vi "From Lockin to Pulse .vi"(7 "Pulse Configuration in":T1={"Post-trigger delay"=0.01, "Post-trigger duration"=0.1, "Rate"=1000000.0, "Ranges"=[10.0], "Re-name channels"=[], "Active channels"="0:1", "External clock"=FALSE} {"Rate" format="%#_8pHz"; "Post-trigger duration" format="%#_6ps"; "Post-trigger delay" format="%#_6ps"; "Ranges" format="%#_6pV"}, 11 "Lockin Configuration in":T2={"Post-trigger delay"=0.01, "Post-trigger duration"=0.1, "Rate"=1000000.0, "Ranges"=[10.0], "Re-name channels"=[], "Active channels"="0:1", "External\nclock"=FALSE, "Frequencies"=[], "Time\nconstant"=1.0, "Output \namplitudes"=[], "Input\nchannles"=[]} {"Output \namplitudes" format="%#_6pV"; "Time\nconstant" format="%#_6ps"; "Frequencies" format="%#_6pHz"; "Rate" format="%#_8pHz"; "Post-trigger duration" format="%#_6ps"; "Post-trigger delay" format="%#_6ps"; "Ranges" format="%#_6pV"}) -> (3 "Pulse  Configuration out":T1={"Post-trigger delay"=0.01, "Post-trigger duration"=0.1, "Rate"=1000000.0, "Ranges"=[10.0], "Re-name channels"=[], "Active channels"="0:1", "External clock"=FALSE} {"Rate" format="%#_8pHz"; "Post-trigger duration" format="%#_6ps"; "Post-trigger delay" format="%#_6ps"; "Ranges" format="%#_6pV"})   [LabVIEW 2021]
uses:
  Pusle Driver Configuration.ctl
  Lockin Digitizer Driver/Lockin Digitizer Configuration.ctl
panel:
  # "Digitizer config"
  # "Lock-in config"
  # "#0\n\n#1"
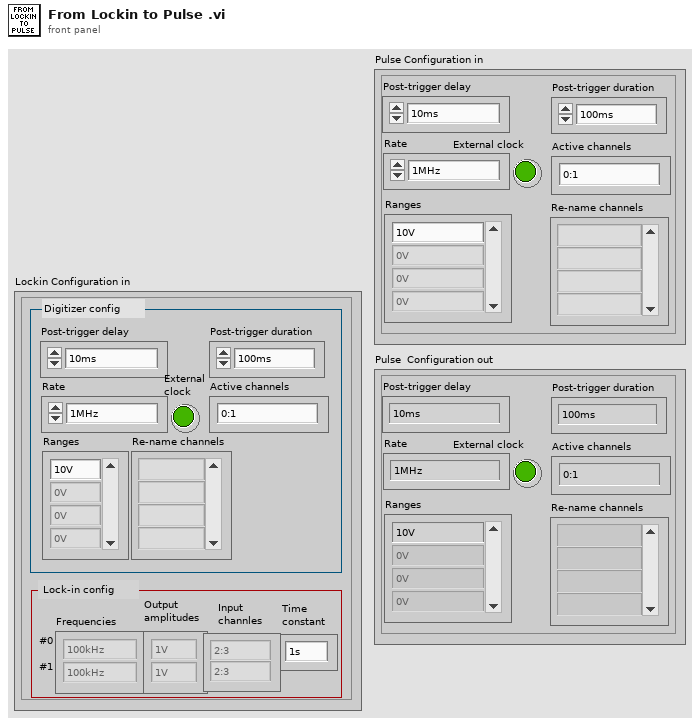
[diagram p1: front panel]
types:
  T1 = typedef "Pusle Driver Configuration.ctl" = cluster{"Post-trigger delay":dbl, "Post-trigger duration":dbl, "Rate":dbl, "Ranges":dbl[], "Re-name channels":string[], "Active channels":string, "External clock":bool}
  T2 = typedef "Lockin Digitizer Configuration.ctl" = cluster{"Post-trigger delay":dbl, "Post-trigger duration":dbl, "Rate":dbl, "Ranges":dbl[], "Re-name channels":string[], "Active channels":string, "External\nclock":bool, "Frequencies":dbl[], "Time\nconstant":dbl, "Output \namplitudes":dbl[], "Input\nchannles":string[]}
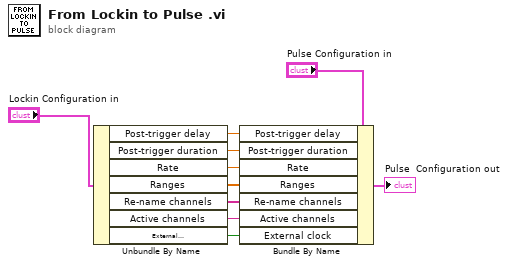
[diagram p0: block diagram]
diagram:
  n1 = Unbundle By Name("Lockin Configuration in") -> ("Post-trigger delay"=w9:dbl, "Post-trigger duration"=w7:dbl, "Rate"=w6:dbl, "Ranges"=w5:dbl[], "Re-name channels"=w4:string[], "Active channels"=w3:string, "External\nclock"=w2:bool)
  n2 = Bundle By Name(cluster="Pulse Configuration in", "Post-trigger delay"=w9, "Post-trigger duration"=w7, "Rate"=w6, "Ranges"=w5, "Re-name channels"=w4, "Active channels"=w3, "External clock"=w2) -> (→"Pulse  Configuration out":T1)
